vi "MeasureJoule.vi"(5 "Junction Name":string, 6 "UiDefinition":T1, 7 ".NET Refnum":refnum<k24>, 8 "new file path (Not A Path if cancelled)":path, 10 "appended path":path, 11 ".NET Refnum in":refnum<k24>) -> (0 "error out":errorcluster, 3 "Cluster":cluster{dbl[], dbl[]})   [LabVIEW 2020]
uses:
  UIReferences.ctl
  D:/LabviewDXFViewer/LabviewDXFViewer/bin/Release/LabviewDXFViewer.exe
  LabviewDXFViewer/bin/Release/LabviewDXFViewer.exe
  <vilib>/Utility/file.llb/Write Delimited Spreadsheet (DBL).vi
  <vilib>/Utility/file.llb/Write Delimited Spreadsheet (string).vi
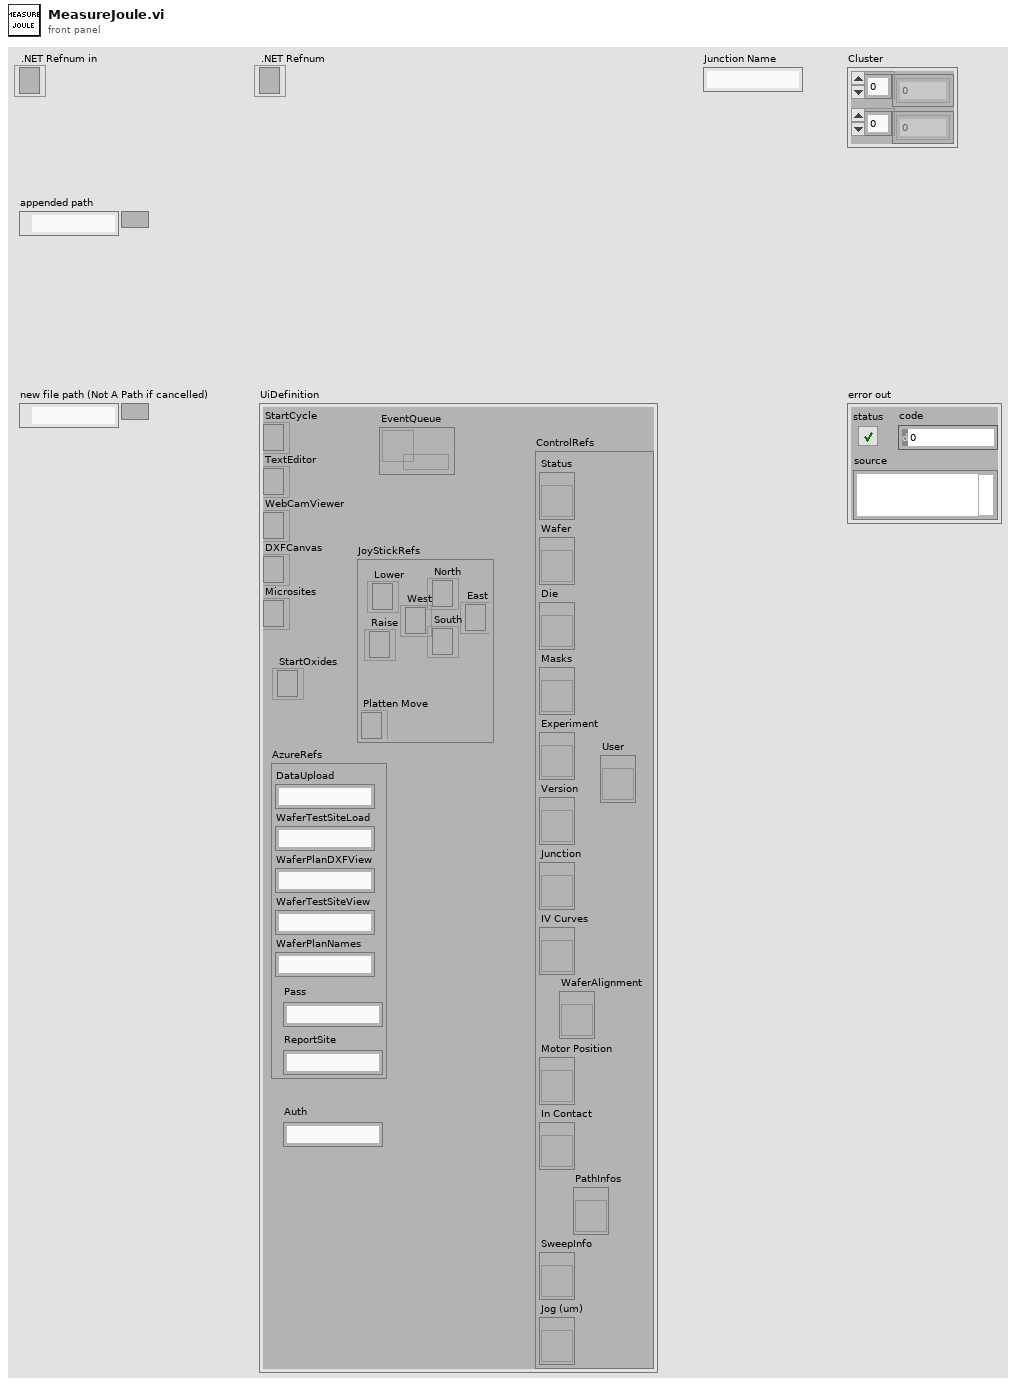
[diagram p1: front panel]
types:
  T1 = typedef "UIReferences.ctl" = cluster{"StartCycle":refnum<k24>, "TextEditor":refnum<k24>, "WebCamViewer":refnum<k24>, "DXFCanvas":refnum<k24>, "Microsites":refnum<k24>, "JoyStickRefs":cluster{"North":refnum<k24>, "Lower":refnum<k24>, "Raise":refnum<k24>, "Platten Move":refnum<k24>, "West":refnum<k24>, "East":refnum<k24>, "South":refnum<k24>}, "AzureRefs":cluster{"DataUpload":string, "WaferTestSiteLoad":string, "WaferPlanDXFView":string, "WaferTestSiteView":string, "WaferPlanNames":string, "Pass":string, "ReportSite":string}, "ControlRefs":cluster{"Status":refnum<vi>, "Wafer":refnum<vi>, "Die":refnum<vi>, "Masks":refnum<vi>, "Experiment":refnum<vi>, "Version":refnum<vi>, "Junction":refnum<vi>, "IV Curves":refnum<vi>, "Motor Position":refnum<vi>, "In Contact":refnum<vi>, "SweepInfo":refnum<vi>, "Jog (um)":refnum<vi>, "PathInfos":refnum<vi>, "User":refnum<vi>, "WaferAlignment":refnum<vi>}, "EventQueue":refnum<queue>, "StartOxides":refnum<k24>, "Auth":string}
  T2 = typedef "CapacitanceInfos.ctl" = cluster{"Conductance":dbl, "CapacitanceIV":dbl, "Intercept":dbl, "CapacitanceSW":dbl, "Sum":dbl, "CapacitanceInfos":T3[], "CapacitancePhase":dbl, "dC/dV":dbl, "Function":string, "OtherInfo":dbl[][]}
  T3 = typedef "CapacitanceRecord.ctl" = cluster{"Freq":dbl, "Vpp":dbl, "PhaseS":dbl, "Irms":dbl, "PhaseC":dbl, "Theta":dbl, "VDrive":dbl, "Capacitance":dbl, "Other":dbl}
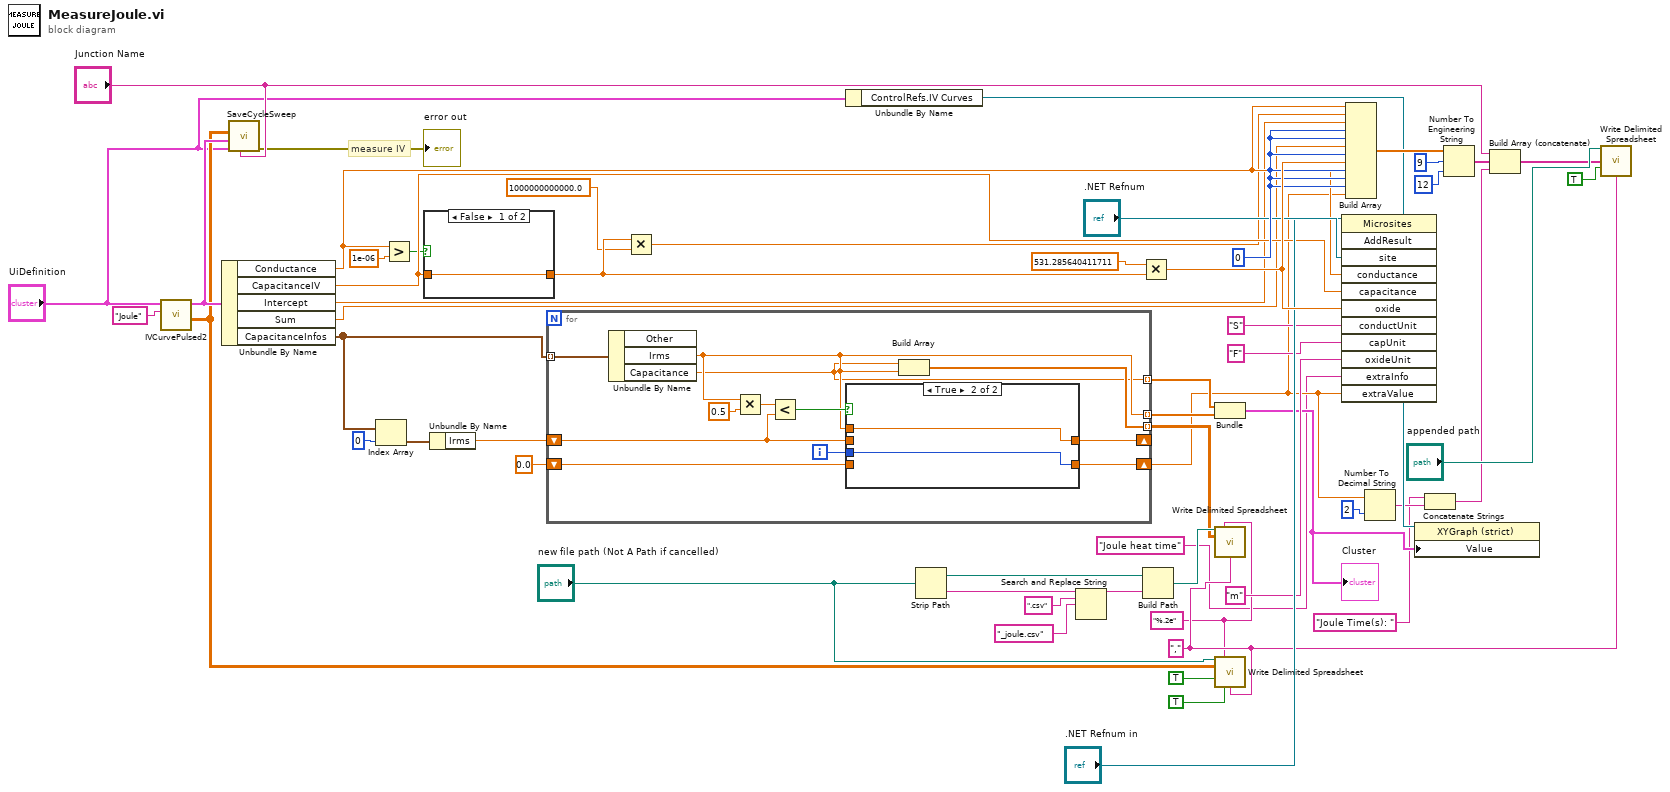
[diagram p0: block diagram]
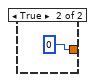
[diagram p3: hidden frame]
diagram:
  w11 = "," ("delimiter (\\t)")
  w54 = 0
  w10 = "%.2e" ("format (%.3f)")
  # "measure IV"
  n1 = call "IVCurvePulsed2.vi"("Program"="Joule", "UiDefinition"="UiDefinition") -> ("appended array"=w27:dbl[][], "InfoCluster"=w40:T2)  [unwired: 8 in]
  n2 = Unbundle By Name(w40) -> ("Conductance"=w42:dbl, "CapacitanceIV"=w41:dbl, "Intercept"=w30:dbl, "Sum"=w31:dbl, "CapacitanceInfos"=w45:T3[])
  n3 = call "SaveCycleSweep.vi"("JunctionName"="Junction Name", "UiDefinition 2"="UiDefinition", "InfoCluster"=w40, "appended array"=w27) -> ("error out"=→"error out":errorcluster)  [unwired: 7 in]
  n4 = Index Array(array=w45, index=0) -> (element=w47:T3)
  n5 = Greater?(x=w42, y=1e-06) -> (0:w34:bool)
  n6 = case shown="False" w34 {
    tunnel: [w58 0] -> w56
    tunnel: w41 -> [w58 _]
    frame False {
    }
    frame True {
    }
  }
  n7 = Unbundle By Name(w47) -> ("Irms"=w48:dbl)
  n8 = for {
    tunnel: w45 -> [w71] mode=indexing
    tunnel: [w60] -> w43 mode=indexing
    tunnel: [w62] -> w44 mode=indexing
    shift-right: [w64] -> _
    shift-left: w48 -> [w65]
    shift-right: [w69] -> w2
    shift-left: 0.0 ("Vpp") -> [w68]
    tunnel: [w61] -> w12 mode=indexing
    i -> [w63]
    n9 = Unbundle By Name(w71) -> ("Irms"=w62:dbl, "Capacitance"=w60:dbl)  [unwired: 1 out]
    n10 = Multiply(x=w62, y=0.5) -> (x*y=w67:dbl)
    n11 = Less?(x=w67, y=w65) -> (x < y?=w70:bool)
    n12 = case shown="True" w70 {
      tunnel: w63 -> [_ w75]
      tunnel: [w73 w75] -> w69
      tunnel: w68 -> [w73 _]
      tunnel: [w72 w74] -> w64
      tunnel: w65 -> [w72 _]
      tunnel: w62 -> [_ w74]
      frame False {
      }
      frame True {
      }
    }
    n13 = Build Array(w60, w62) -> (w61:dbl[])
  }
  n14 = Multiply(x=w56, y=1000000000000.0) -> (x*y=w32:dbl)
  n15 = Unbundle By Name("UiDefinition") -> ("ControlRefs.IV Curves"=w8:refnum<vi>)
  n16 = Strip Path(path="new file path (Not A Path if cancelled)") -> (stripped path=w15:path, name=w19:string)
  n17 = Search and Replace String(input string=w19, search string=".csv", replace string="_joule.csv" ("replace string (\"\")")) -> (result string=w16:string)  [unwired: 5 in, 3 out]
  n18 = Multiply(x=531.285640411711, y=w56) -> (x*y=w57:dbl)
  n19 = Build Path(base path=w15, name or relative path=w16) -> (appended path=w13:path)
  n20 = Bundle(w43, w44) -> (w7:cluster{dbl[], dbl[]})  [unwired: 1 in]
  "Cluster" <- w7
  n21 = call-poly <vilib>:"Write Delimited Spreadsheet.vi"("file path (dialog if empty)"=w13, "format (%.3f)"=w10, "2D data"=w12, "delimiter (\\t)"=w11) -> ()  [unwired: 10 in, 2 out]
  n22 = call-poly <vilib>:"Write Delimited Spreadsheet.vi"("file path (dialog if empty)"="new file path (Not A Path if cancelled)", "format (%.3f)"=w10, "2D data"=w27, "append to file? (new file:F)"=TRUE, "transpose? (no:F)"=TRUE, "delimiter (\\t)"=w11) -> ()  [unwired: 8 in, 2 out]
  n23 = invoke class="Microsites" method="AddResult"(reference=".NET Refnum in", "site"=".NET Refnum", "conductance"=w42, "capacitance"=w41, "oxide"=w57, "conductUnit"="S", "capUnit"="F", "oxideUnit"="m" ("interceptUnit"), "extraInfo"="Joule heat time", "extraValue"=w2) -> ()  [unwired: 2 in, 12 out]
  n24 = Build Array(w42, w32, w30, w54, w54, w31, w54, w57, w54, w54, w54, w2) -> (w29:dbl[])
  n25 = Number To Decimal String(number=w2, width (-)=i16 2) -> (decimal integer string=w6:string)
  n26 = property class="XYGraph (strict)"(reference=w8, "Value"=w7) -> ()  [unwired: 1 in, 2 out]
  n27 = Concatenate Strings("Joule Time(s): ", w6) -> (w3:string)
  n28 = Number To Engineering String(2:i16 12 ("precision (6)"), 3:i16 9 ("width (-)"), 4:w29) -> (0:w22:string[])  [unwired: 1 in]
  n29 = Build Array (concatenate)("Junction Name", w22, w3) -> (w24:string[])
  n30 = call-poly <vilib>:"Write Delimited Spreadsheet.vi"("file path (dialog if empty)"="appended path", "1D data"=w24, "append to file? (new file:F)"=TRUE, "delimiter (\\t)"=w11) -> ()  [unwired: 10 in, 2 out]
